vi "copy - Vector Copy.vi"   [LabVIEW 2014, in "NI_AALBLAS.lvlib"]
doc: "Replaces elements in <B>y</B> with elements in <B>x</B>."
uses:
  NI_AALBLAS.lvlib
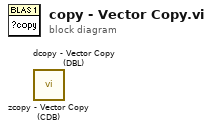
[diagram p0: block diagram]
diagram:
  n1 = call "zcopy - Vector Copy (CDB).vi"() -> ()  [unwired: 10 in, 2 out]
  n2 = call "dcopy - Vector Copy (DBL).vi"() -> ()  [unwired: 10 in, 2 out]
